vi "readADC.vi"(7 "x(0), y(0)":fxp<+/-,16,5>[](array[numeric]), 8 "z-height":refnum<k21>="Mod2/AI3", 9 "z-err- ADC":refnum<k21>="Mod2/AI2", 10 "y - ADC":refnum<k21>="Mod2/AI1", 11 "x - ADC":refnum<k21>="Mod2/AI0") -> (2 "x_y_ze_z_k":fxp<+/-,17,6>[](array[numeric]))   [LabVIEW 2017]
uses:
  <vilib>/rvi/eio/common/nirviEmuTemplateMethod_errors.vi
  <vilib>/eio/EIONode/EIONode.xnode
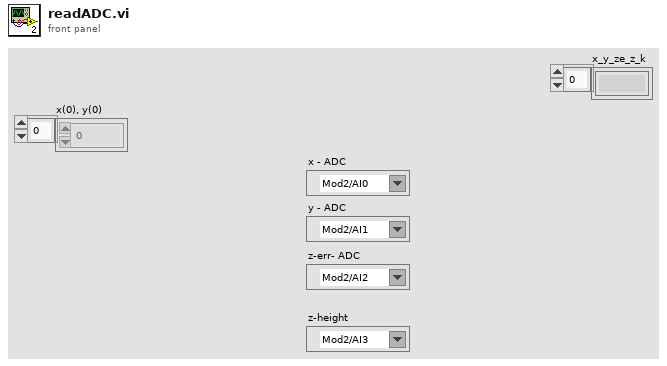
[diagram p1: front panel]
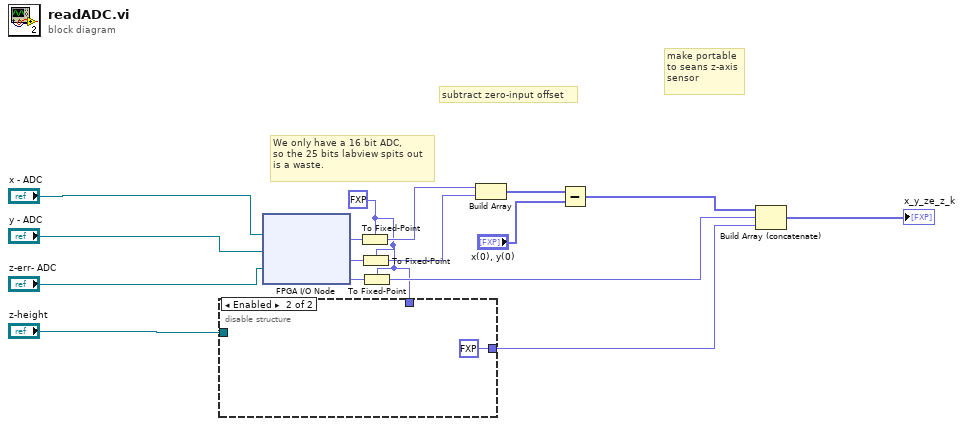
[diagram p0: block diagram]
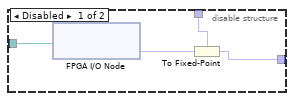
[diagram p2: hidden frame]
diagram:
  w1 = fxp<+/-,16,5> 0.0 ("fixed-point type")
  # "We only have a 16 bit ADC,\nso the 25 bits labview spits out\nis a waste."
  # "make portable\nto seans z-axis\nsensor"
  # "subtract zero-input offset"
  n1 = disable-structure shown="Enabled" {
    disable-tunnel: "z-height" -> [w20 _]
    disable-tunnel: [w18 fxp<+/-,16,5> 0.0] -> w8
    disable-tunnel: w1 -> [w17 _]
    frame Disabled {
      n2 = xnode "FPGA I/O Node"("FPGA I/O In"=w20) -> ("I/O Item"=w19:fxp<+/-,24,5>)  [unwired: 1 out]
      n3 = To Fixed-Point(fixed-point type=w17, number=w19) -> (fixed-point=w18:fxp<+/-,16,5>)
    }
    frame Enabled {
    }
  }
  n4 = xnode "FPGA I/O Node"("FPGA I/O In"="x - ADC", "FPGA I/O In"="y - ADC", "FPGA I/O In"="z-err- ADC") -> ("I/O Item"=w7:fxp<+/-,24,5>, "I/O Item"=w5:fxp<+/-,24,5>, "I/O Item"=w3:fxp<+/-,24,5>)  [unwired: 3 out]
  n5 = To Fixed-Point(fixed-point type=w1, number=w7) -> (fixed-point=w6:fxp<+/-,16,5>)
  n6 = To Fixed-Point(fixed-point type=w1, number=w5) -> (fixed-point=w4:fxp<+/-,16,5>)
  n7 = To Fixed-Point(fixed-point type=w1, number=w3) -> (fixed-point=w2:fxp<+/-,16,5>)
  n8 = Build Array(w6, w4) -> (w15:fxp<+/-,16,5>[])
  n9 = Subtract(x=w15, y="x(0), y(0)") -> (x-y=w13:fxp<+/-,17,6>[])
  n10 = Build Array (concatenate)(w13, w2, w8) -> (→"x_y_ze_z_k":fxp<+/-,17,6>[])
